vi "logon enviro tcp.vi"(8 "error in":errorcluster) -> (0 "error out":errorcluster, 2 "data server address":string="128.84.245.239", 3 "connection ID":refnum<k5>)   [LabVIEW 2010]
doc: "Open data server opens a connection with a data server. If the array of data servers contains only one element then the connection is made immediately. If the array contains more than one element a subvi with a dialog box opens to select the data server. TCP is then used to log on to the data server and data server information is returned in the Server Stats control.\n\nInputs\n\nPort - TCP port number. Must be the same as the port number used by the data server. At Cornell CEE we use port 6341.\n\nData Servers - An array of strings that are either names or IP addresses for available dataservers \n\nError in - \n\nOutputs\n\nData server address - String containing the name or the IP address of the selected data server.\n\nRestart - Boolean that is true if the connection with the data server could not be established.\n\nServer Stats - Data server information including scan rate, number of client connections and channel information.\n\nError out - \n\n\nCreated by Monroe Weber-Shirk\nCornell University\nmw24@cornell.edu\nJanuary 2000"
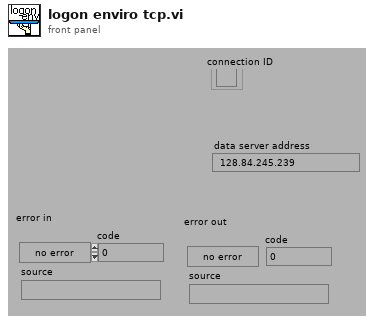
[diagram p1: front panel]
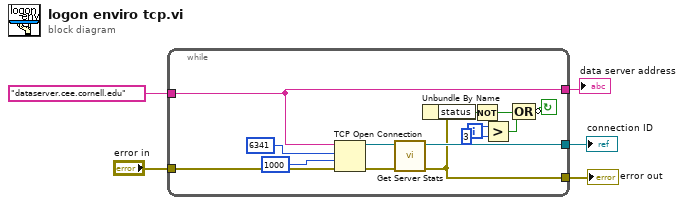
[diagram p0: block diagram]
diagram:
  n1 = while {
    tunnel: "dataserver.cee.cornell.edu" -> [w6]
    tunnel: "error in" -> [w13]
    tunnel: [w14] -> w3
    tunnel: [w17] -> w4
    tunnel: [w6] -> w5
    i -> [w10]
    stop <- w12 continue-if-true
    n2 = TCP Open Connection(address=w6, remote port or service name=u16 6341 ("port"), timeout ms (60000)=1000, error in (no error)=w13) -> (connection ID=w18:refnum<k5>, error out=w19:errorcluster)  [unwired: 1 in]
    n3 = call "Get Server Stats.vi"("error in (no error)"=w19, "Connection ID"=w18) -> ("error out"=w14:errorcluster, "Connection ID"=w17:refnum<k5>)  [unwired: 6 in, 2 out]
    n4 = Unbundle By Name(w14) -> ("status"=w15:bool)
    n5 = Not(x=w15) -> (.not. x?=w11:bool)
    n6 = Greater?(x=w10, y=3) -> (0:w8:bool)
    n7 = Compound Arithmetic op=OR(w11, w8) -> (invert w12:bool)
  }
  "data server address" <- w5
  "connection ID" <- w4
  "error out" <- w3
